vi "FormElecHouseRawCmd.vi"(7 "Preamble":string="UU\u0000\u0000\u0000", 11 "Command":string="Ô@\u00010\u0004") -> (4 "concatenated Cmd":string)   [LabVIEW 2012, in "NFC Driver.lvlib"]
doc: "This VI formats the string specified by \"Command\" and formats it into a PN532 command according to UM0701-02 (PN532 User Manual Rev. 2).\n\nThe format is as follows:\nB1 - Preamble\nB2,B3 - Start of command\nB4 - Command Length\nB5 - Length checksum\nB6,B7...Bn - Command\nBn+1 - Command checksum\nBn+2 - Postamble"
uses:
  NFC Driver.lvlib
panel:
  out "DCS":i8 format="%x"
  out "LCS":u8 format="%x"
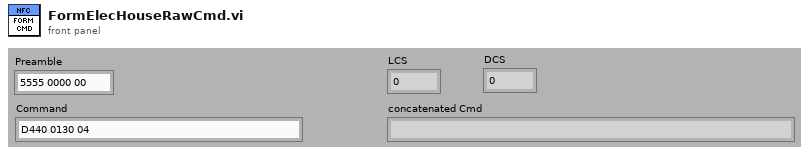
[diagram p1: front panel]
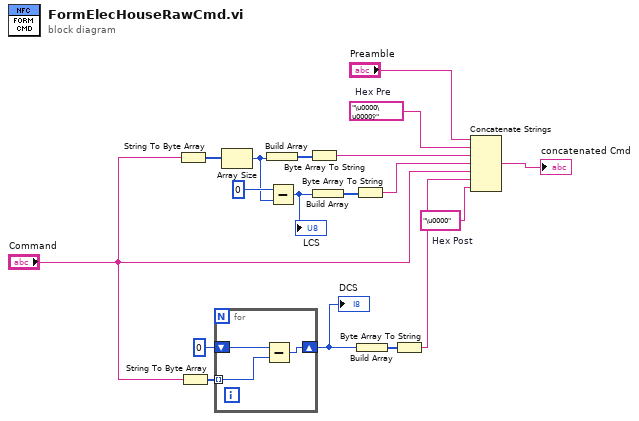
[diagram p0: block diagram]
diagram:
  w2 = "\u0000\u0000ÿ"  # Hex Pre
  w4 = "\u0000"  # Hex Post
  n1 = String To Byte Array(string="Command") -> (unsigned byte array=w18:u8[])
  n2 = String To Byte Array(string="Command") -> (unsigned byte array=w6:u8[])
  n3 = for {
    tunnel: w6 -> [w20] mode=indexing
    shift-right: [w21] -> w8
    shift-left: u8 0 -> [w19]
    n4 = Subtract(x=w19, y=w20) -> (x-y=w21:u8)
  }
  "DCS" <- w8
  n5 = Array Size(array=w18) -> (size(s)=w15:i32)
  n6 = Build Array(w15) -> (w17:i32[])
  n7 = Subtract(x=0 ("y"), y=w15) -> (x-y=w13:i32)
  "LCS" <- w13
  n8 = Byte Array To String(unsigned byte array=w17) -> (string=w12:string)
  n9 = Build Array(w13) -> (w14:i32[])
  n10 = Byte Array To String(unsigned byte array=w14) -> (string=w11:string)
  n11 = Build Array(w8) -> (w9:u8[])
  n12 = Byte Array To String(unsigned byte array=w9) -> (string=w5:string)
  n13 = Concatenate Strings("Preamble", w2, w12, w11, "Command", w5, w4) -> (→"concatenated Cmd":string)
